vi "Deadzone.vi"(2 "Deadzone":dbl, 3 "Value":dbl) -> (0 "Inside Deadzone?":bool, 1 "Numeric":dbl)   [LabVIEW 2018, in "Huskie Swerve.lvlib"]
uses:
  HuskieLibrary/SwerveLibrary--need to sort/Huskie Swerve.lvlib
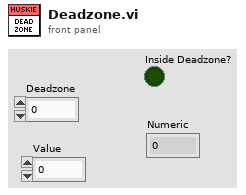
[diagram p1: front panel]
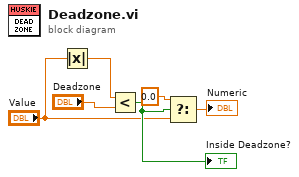
[diagram p0: block diagram]
diagram:
  n1 = Absolute Value(x="Value") -> (abs(x)=w4:dbl)
  n2 = Less?(x=w4, y="Deadzone") -> (x < y?=w5:bool)
  "Inside Deadzone?" <- w5
  n3 = Select(t=0.0, s=w5, f="Value") -> (s? t:f=→"Numeric":dbl)
